vi "ThreeIncoming.vi"() -> ()   [LabVIEW 2019]
uses:
  <vilib>/rvi/Emulation/niFpgaGetClockAttributes.vi
  <vilib>/rvi/Emulation/niFpgaSctlEmulationGetInTimedLoop.vi
  <vilib>/rvi/Emulation/niFpgaEmulationReportErrorSimple.vi
  <vilib>/rvi/Emulation/niFpgaCriticalErrorInLSC.vi
  <vilib>/rvi/interface/RandomDataEmulation/niFpgaRandomDataHandleErrors.vi
  <vilib>/rvi/DataTransferAndStorage/Container/XNode/niFpgaContainer.xnode
  <vilib>/rvi/interface/RandomDataEmulation/nirviRandomDataFpgaReadWriteTemplate.vi
  <vilib>/Platform/TimedLoop/XDataNode/wakeup.ctl
  <vilib>/Platform/TimedLoop/XDataNode/XDNodeRunTimeDep.lvlib
  <vilib>/Platform/TimedLoop/XDataNode/nitl_modes.ctl
  <vilib>/Platform/TimedLoop/XDataNode/timing_clust.ctl
  <vilib>/Platform/TimedLoop/XDataNode/XDataNode.xnode
  SubModules/FPGA Addon Speciality IO/Source/Speciality FPGA IO.lvlib
  SubModules/FPGA Addon Speciality IO/Source/Types/QuadratureEncoder.Measure.Digital.Settings.ctl
  SubModules/FPGA Addon Speciality IO/Source/Types/QuadratureEncoder.Measure.Digital.Measurement.ctl
  SubModules/FPGA Addon Speciality IO/Source/Types/WSS.Generate.Digital.Settings.ctl
  SubModules/FPGA Addon Speciality IO/Source/Types/Static.Measure.Digital.Measurement.ctl
  SubModules/FPGA Addon Speciality IO/Source/Types/Static.Measure.Digital.Settings.ctl
  SubModules/FPGA Addon Speciality IO/Source/Types/Static.Generate.Digital.Settings.ctl
  SubModules/FPGA Addon Speciality IO/Source/Types/PWM.Generate.Digital.Settings.ctl
  SubModules/FPGA Addon Speciality IO/Source/Types/PWM.Measure.Digital.Settings.ctl
  SubModules/FPGA Addon Speciality IO/Source/Types/PWM.Measure.Digital.Measurement.ctl
panel:
  out "Measure.Digital.Ch0":T1={"ACTIVE TICKS"=4000, "INACTIVE TICKS"=12000, "ACQ TICKS"=1}
  out "Measure.Digital.Ch1":T1
  in  "Measure.Digital.Ch0.Settings":T2={"ACTIVE EDGE"=TRUE, "TIMEOUT"=40000000}
  in  "Measure.Digital.Ch1.Settings":T2={"ACTIVE EDGE"=FALSE, "TIMEOUT"=40000000}
  in  "Generate.Digital.Ch0.Internal.Settings":T3={"ACTIVE EDGE"=TRUE, "ACTIVE TICKS"=4000, "INACTIVE TICKS"=12000}
  in  "Generate.Digital.Ch1.Internal.Settings":T3={"ACTIVE EDGE"=FALSE, "ACTIVE TICKS"=60000000, "INACTIVE TICKS"=20000000}
  in  "Generate.Digital.Ch2.Internal.Settings":T4={"ACTIVE EDGE"=TRUE, "OUTPUT"=FALSE}
  in  "Measure.Digital.Ch2.Internal.Settings":T5={"ACTIVE EDGE"=TRUE}
  out "Measure.Digital.Ch2":T6
  in  "Generate.Digital.Ch3.Internal.Settings":T4={"ACTIVE EDGE"=TRUE, "OUTPUT"=FALSE}
  in  "Measure.Digital.Ch3.Internal.Settings":T5={"ACTIVE EDGE"=TRUE}
  out "Measure.Digital.Ch3":T6
  in  "Generate.Digital.Ch4.WSS.Settings":T7={"ACTIVE EDGE"=TRUE, "ACTIVE TICKS"=0, "INACTIVE TICKS"=0, "DATA"=0, "SENSOR TYPE"=0}
  out "Bit0":bool
  out "Bit1":bool
  out "Measurement.Digital.Ch5":T8
  in  "A":bool
  in  "B":bool
  in  "Z":bool
  in  "Measure.Digital.Ch5.QuadEncoder.Settings":T9={"DIRECTION"=0, "RESET VALUE"=0, "A RESET STATE"=TRUE, "B RESET STATE"=TRUE, "Z RESET STATE"=TRUE}
  in  "Group1.I16":i16
  in  "Group1.I8":i8
  in  "Group1.I64":i64
  in  "Group1.I32":i32
  in  "Group1.U16":u16
  in  "Group1.U8":u8
  in  "Group1.U64":u64
  in  "Group1.U32":u32
  in  "Group1.SGL":sgl
  in  "Group2.Boolean":bool
  out "Group1.I16 out":i16
  out "Group1.I8 out":i8
  out "Group1.I64 out":i64
  out "Group1.I32 out":i32
  out "Group1.U16 out":u16
  out "Group1.U8 out":u8
  out "Group1.U64 out":u64
  out "Group1.U32 out":u32
  out "Group1.SGL out":sgl
  out "Group2.Boolean out":bool
  in  "Group2.FXP24.5":fxp<+/-,24,5>
  in  "Group2.FXP16.5":fxp<+/-,16,5>
  in  "Group2.FXP32.8":fxp<+/-,32,8>
  in  "Group2.FXP64.32":fxp<+/-,64,32>
  out "Group2.FXP24.5 out":fxp<+/-,24,5>
  out "Group2.FXP16.5 out":fxp<+/-,16,5>
  out "Group2.FXP32.8 out":fxp<+/-,32,8>
  out "Group2.FXP64.32 out":fxp<+/-,64,32>
  in  "Group2.FXP16.7":fxp<+/-,16,7>
  out "Group2.FXP16.7 out":fxp<+/-,16,7>
  in  "Group2.FXP20.5":fxp<+/-,20,5>
  out "Group2.FXP20.5 out":fxp<+/-,20,5>
  in  "Group2.FXP27.5":fxp<+/-,27,5>
  out "Group2.FXP27.5 out":fxp<+/-,27,5>
  in  "Group2.FXP32.16":fxp<+/-,32,16>
  out "Group2.FXP32.16 out":fxp<+/-,32,16>
  in  "Group2.FXP16.3":fxp<+,16,3>
  out "Group2.FXP16.3 out":fxp<+,16,3>
  in  "Group2.FXP18.3":fxp<+,18,3>
  out "Group2.FXP18.3 out":fxp<+,18,3>
  in  "FXP18.3":fxp<+,18,3>
  out "FXP18.3 out":fxp<+,18,3>
  in  "FXP16.3":fxp<+,16,3>
  out "FXP16.3 out":fxp<+,16,3>
  in  "FXP32.16":fxp<+/-,32,16>
  out "FXP32.16 out":fxp<+/-,32,16>
  in  "FXP27.5":fxp<+/-,27,5>
  out "FXP27.5 out":fxp<+/-,27,5>
  in  "FXP20.5":fxp<+/-,20,5>
  out "FXP20.5 out":fxp<+/-,20,5>
  in  "FXP16.7":fxp<+/-,16,7>
  out "FXP16.7 out":fxp<+/-,16,7>
  out "FXP64.32 out":fxp<+/-,64,32>
  out "FXP32.8 out":fxp<+/-,32,8>
  out "FXP16.5 out":fxp<+/-,16,5>
  out "FXP24.5 out":fxp<+/-,24,5>
  in  "FXP64.32":fxp<+/-,64,32>
  in  "FXP32.8":fxp<+/-,32,8>
  in  "FXP16.5":fxp<+/-,16,5>
  in  "FXP24.5":fxp<+/-,24,5>
  out "Fast timeout":bool
  out "Med timeout":bool
  out "Slow timeout":bool
  in  "I16":i16
  in  "I8":i8
  in  "I64":i64
  in  "I32":i32
  in  "U16":u16
  in  "U8":u8
  in  "U64":u64
  in  "U32":u32
  in  "SGL":sgl
  in  "Boolean":bool
  out "I16 out":i16
  out "I8 out":i8
  out "I64 out":i64
  out "I32 out":i32
  out "U16 out":u16
  out "U8 out":u8
  out "U64 out":u64
  out "U32 out":u32
  out "SGL out":sgl
  out "Boolean out":bool
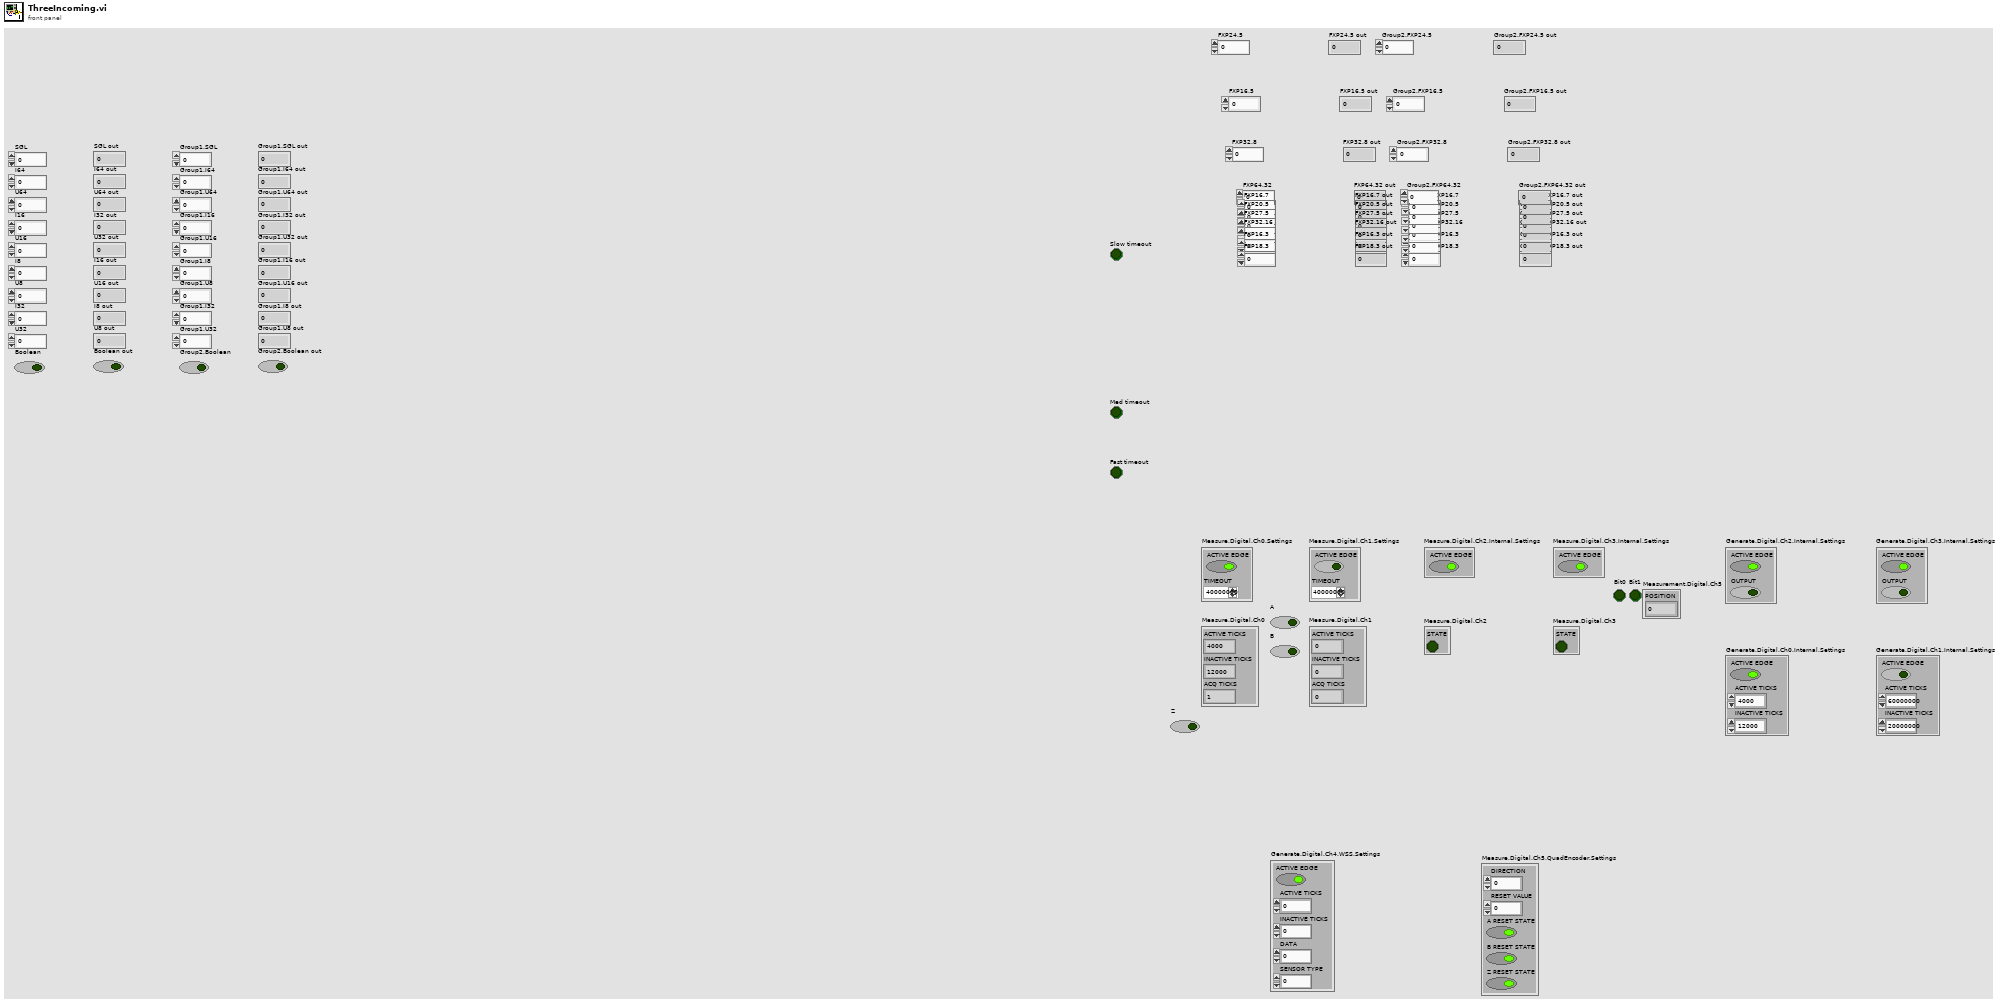
[diagram p1: front panel]
types:
  T1 = typedef "Speciality FPGA IO.lvlib/PWM.Measure.Digital.Measurement.ctl" = cluster{"ACTIVE TICKS":u32, "INACTIVE TICKS":u32, "ACQ TICKS":u32}
  T2 = typedef "Speciality FPGA IO.lvlib/PWM.Measure.Digital.Settings.ctl" = cluster{"ACTIVE EDGE":bool, "TIMEOUT":u32}
  T3 = typedef "Speciality FPGA IO.lvlib/PWM.Generate.Digital.Settings.ctl" = cluster{"ACTIVE EDGE":bool, "ACTIVE TICKS":u32, "INACTIVE TICKS":u32}
  T4 = typedef "Speciality FPGA IO.lvlib/Static.Generate.Digital.Settings.ctl" = cluster{"ACTIVE EDGE":bool, "OUTPUT":bool}
  T5 = typedef "Speciality FPGA IO.lvlib/Static.Measure.Digital.Settings.ctl" = cluster{"ACTIVE EDGE":bool}
  T6 = typedef "Speciality FPGA IO.lvlib/Static.Measure.Digital.Measurement.ctl" = cluster{"STATE":bool}
  T7 = typedef "Speciality FPGA IO.lvlib/WSS.Generate.Digital.Settings.ctl" = cluster{"ACTIVE EDGE":bool, "ACTIVE TICKS":u32, "INACTIVE TICKS":u32, "DATA":u8, "SENSOR TYPE":u8}
  T8 = typedef "Speciality FPGA IO.lvlib/QuadratureEncoder.Measure.Digital.Measurement.ctl" = cluster{"POSITION":i32}
  T9 = typedef "Speciality FPGA IO.lvlib/QuadratureEncoder.Measure.Digital.Settings.ctl" = cluster{"DIRECTION":u8, "RESET VALUE":i32, "A RESET STATE":bool, "B RESET STATE":bool, "Z RESET STATE":bool}
  T10 = typedef "XDNodeRunTimeDep.lvlib/timing_clust.ctl" = cluster{"Expected End [f-1]":u64, "Actual End [f-1]":u64, "Finished Late? [f-1]":bool, "Expected End [i-1]":u64, "Actual End [i-1]":u64, "Finished Late? [i-1]":bool, "Expected Start [i]":u64, "Actual Start [i]":u64, "Expected Start [f]":u64, "Actual Start [f]":u64, "Source Name":string, "Structure Name":string, "Period":i64, "Deadline":i64, "Offset":i64, "Start":i64, "Priority":i32, "Timeout":i32, "Mode":T11, "Wakeup Reason":T12, "Error":errorcluster, "Source Type":string, "Secondary Source Type":string, "Global End Time":u64, "Global Start Time":u64, "Frame Duration":u64, "Iteration Duration":u64, "Assigned CPU":i32, "I/O Scan Engine Mode":u32}
  T11 = typedef "XDNodeRunTimeDep.lvlib/nitl_modes.ctl" = enum32{"No Change", "Process missed periods, maintain original phase", "Discard missed periods, maintain original phase", "Process missed periods, ignore original phase", "Discard missed periods, ignore original phase"}
  T12 = typedef "XDNodeRunTimeDep.lvlib/wakeup.ctl" = enum32{"Normal", "Aborted", "Asynchronous wakeup", "Timing source error", "Timed loop error", "Timeout"}
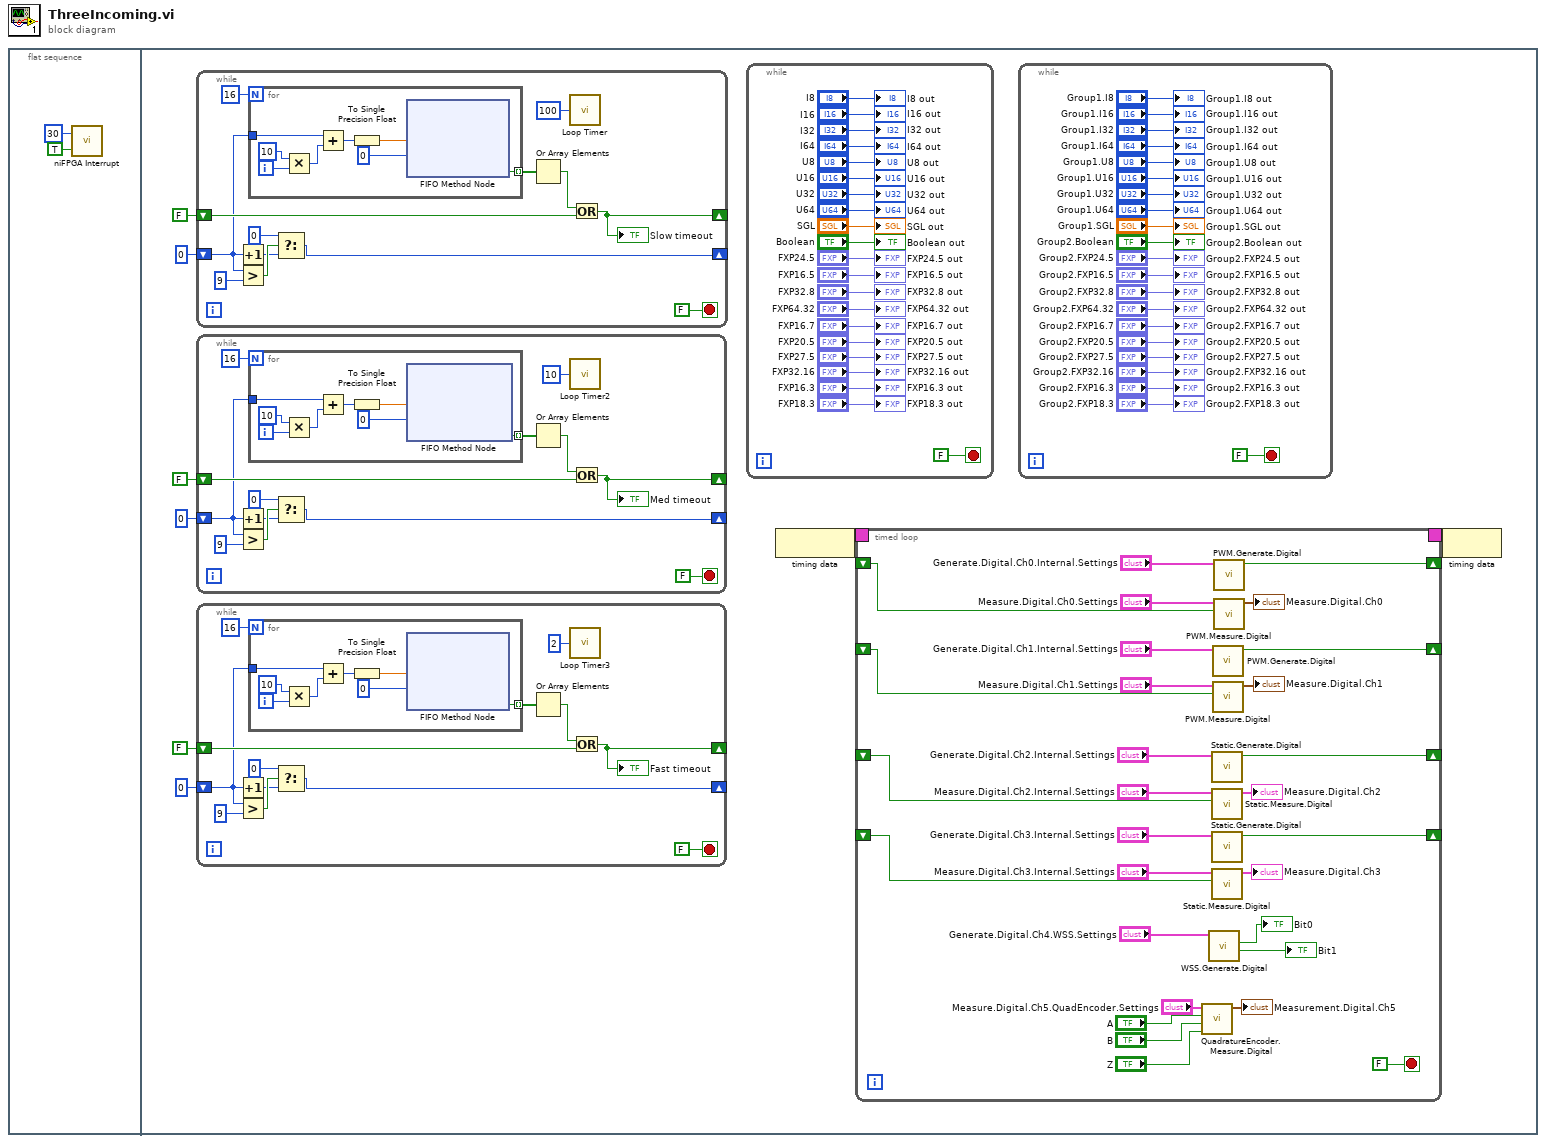
[diagram p0: block diagram]
diagram:
  n1 = flat-sequence {
    frame #0 {
      n2 = call <vilib>:"niFPGA Interrupt.vi"("Wait Until Cleared (F)"=TRUE, "IRQ Number (0)"=u8 30) -> ()  [unwired: 1 in]
    }
    frame #1 {
      n3 = while {
        shift-right: [w114] -> _
        shift-left: 0 ("t") -> [w107]
        shift-right: [w108] -> _
        shift-left: FALSE -> [w109]
        stop <- FALSE stop-if-true
        n4 = Increment(x=w107) -> (x+1=w112:i32)
        n5 = Greater?(x=w107, y=9) -> (0:w118:bool)
        n6 = for {
          N: 16 -> [_]
          tunnel: w107 -> [w127]
          tunnel: [w120] -> w111 mode=indexing
          i -> [w126]
          n7 = Multiply(x=10, y=w126) -> (x*y=w124:i32)
          n8 = Add(x=w127, y=w124) -> (x+y=w123:i32)
          n9 = To Single Precision Float(number=w123) -> (single precision float=w122:sgl)
          n10 = xnode ("FIFO Method Node")("Element"=w122, "Timeout"=0) -> ("Timed Out?"=w120:bool)  [unwired: 1 in, 1 out]
        }
        n11 = Select(t=0, s=w118, f=w112) -> (s? t:f=w114:i32)
        n12 = Or Array Elements(Boolean array=w111) -> (logical OR=w110:bool)
        n13 = call "Loop Timer"("Count(uSec)"=u32 100) -> ()  [unwired: 1 out]
        n14 = Or(x=w110, y=w109) -> (x .or. y?=w108:bool)
        "Slow timeout" <- w108
      }
      n15 = while {
        shift-right: [w93] -> _
        shift-left: 0 ("t") -> [w86]
        shift-right: [w87] -> _
        shift-left: FALSE -> [w88]
        stop <- FALSE stop-if-true
        n16 = Increment(x=w86) -> (x+1=w91:i32)
        n17 = Greater?(x=w86, y=9) -> (0:w97:bool)
        n18 = for {
          N: 16 -> [_]
          tunnel: w86 -> [w106]
          tunnel: [w99] -> w90 mode=indexing
          i -> [w105]
          n19 = Multiply(x=10, y=w105) -> (x*y=w103:i32)
          n20 = Add(x=w106, y=w103) -> (x+y=w102:i32)
          n21 = To Single Precision Float(number=w102) -> (single precision float=w101:sgl)
          n22 = xnode ("FIFO Method Node")("Element"=w101, "Timeout"=0) -> ("Timed Out?"=w99:bool)  [unwired: 1 in, 1 out]
        }
        n23 = Select(t=0, s=w97, f=w91) -> (s? t:f=w93:i32)
        n24 = Or Array Elements(Boolean array=w90) -> (logical OR=w89:bool)
        n25 = call "Loop Timer2"("Count(uSec)"=u32 10) -> ()  [unwired: 1 out]
        n26 = Or(x=w89, y=w88) -> (x .or. y?=w87:bool)
        "Med timeout" <- w87
      }
      n27 = while {
        shift-right: [w72] -> _
        shift-left: 0 ("t") -> [w65]
        shift-right: [w66] -> _
        shift-left: FALSE -> [w67]
        stop <- FALSE stop-if-true
        n28 = Increment(x=w65) -> (x+1=w70:i32)
        n29 = Greater?(x=w65, y=9) -> (0:w76:bool)
        n30 = for {
          N: 16 -> [_]
          tunnel: w65 -> [w85]
          tunnel: [w78] -> w69 mode=indexing
          i -> [w84]
          n31 = Multiply(x=10, y=w84) -> (x*y=w82:i32)
          n32 = Add(x=w85, y=w82) -> (x+y=w81:i32)
          n33 = To Single Precision Float(number=w81) -> (single precision float=w80:sgl)
          n34 = xnode ("FIFO Method Node")("Element"=w80, "Timeout"=0) -> ("Timed Out?"=w78:bool)  [unwired: 1 in, 1 out]
        }
        n35 = Select(t=0, s=w76, f=w70) -> (s? t:f=w72:i32)
        n36 = Or Array Elements(Boolean array=w69) -> (logical OR=w68:bool)
        n37 = call "Loop Timer3"("Count(uSec)"=u32 2) -> ()  [unwired: 1 out]
        n38 = Or(x=w68, y=w67) -> (x .or. y?=w66:bool)
        "Fast timeout" <- w66
      }
      n39 = while {
        stop <- FALSE stop-if-true
        "I16 out" <- "I16"
        "I8 out" <- "I8"
        "I64 out" <- "I64"
        "I32 out" <- "I32"
        "U16 out" <- "U16"
        "U8 out" <- "U8"
        "U64 out" <- "U64"
        "U32 out" <- "U32"
        "SGL out" <- "SGL"
        "Boolean out" <- "Boolean"
        "FXP24.5 out" <- "FXP24.5"
        "FXP16.5 out" <- "FXP16.5"
        "FXP32.8 out" <- "FXP32.8"
        "FXP64.32 out" <- "FXP64.32"
        "FXP16.7 out" <- "FXP16.7"
        "FXP20.5 out" <- "FXP20.5"
        "FXP27.5 out" <- "FXP27.5"
        "FXP32.16 out" <- "FXP32.16"
        "FXP16.3 out" <- "FXP16.3"
        "FXP18.3 out" <- "FXP18.3"
      }
      n40 = node-c288() -> (w4:T10)
      n41 = timed-loop {
        timing: w4 -> [_]
        timing-out: [_] -> w3
        shift-right: [w38] -> _
        shift-left: _ -> [w37]
        shift-right: [w36] -> _
        shift-left: _ -> [w35]
        shift-right: [w28] -> _
        shift-left: _ -> [w26]
        shift-right: [w19] -> _
        shift-left: _ -> [w21]
        stop <- FALSE stop-if-true
        n42 = call "QuadratureEncoder.Measure.Digital.vi"("Z"="Z", "B"="B", "A"="A", "Settings"="Measure.Digital.Ch5.QuadEncoder.Settings") -> ("Measurement"=→"Measurement.Digital.Ch5":T8)  [unwired: 7 in]
        n43 = call "WSS.Generate.Digital.vi"("Settings"="Generate.Digital.Ch4.WSS.Settings") -> ("Bit1"=→"Bit1":bool, "Bit0"=→"Bit0":bool)  [unwired: 8 in, 1 out]
        n44 = call "Static.Generate.Digital.vi"("Settings"="Generate.Digital.Ch2.Internal.Settings") -> ("Output"=w28:bool)  [unwired: 10 in]
        n45 = call "Static.Measure.Digital.vi"("State"=w26, "Settings"="Measure.Digital.Ch2.Internal.Settings") -> ("Measurement"=→"Measure.Digital.Ch2":T6)  [unwired: 9 in]
        n46 = call "Static.Generate.Digital.vi"("Settings"="Generate.Digital.Ch3.Internal.Settings") -> ("Output"=w19:bool)  [unwired: 10 in]
        n47 = call "Static.Measure.Digital.vi"("State"=w21, "Settings"="Measure.Digital.Ch3.Internal.Settings") -> ("Measurement"=→"Measure.Digital.Ch3":T6)  [unwired: 9 in]
        n48 = call "PWM.Generate.Digital.vi"("Settings"="Generate.Digital.Ch1.Internal.Settings") -> ("Output"=w38:bool)  [unwired: 10 in]
        n49 = call "PWM.Measure.Digital.vi"("State"=w37, "Settings"="Measure.Digital.Ch1.Settings") -> ("Measurement"=→"Measure.Digital.Ch1":T1)  [unwired: 8 in, 1 out]
        n50 = call "PWM.Generate.Digital.vi"("Settings"="Generate.Digital.Ch0.Internal.Settings") -> ("Output"=w36:bool)  [unwired: 10 in]
        n51 = call "PWM.Measure.Digital.vi"("State"=w35, "Settings"="Measure.Digital.Ch0.Settings") -> ("Measurement"=→"Measure.Digital.Ch0":T1)  [unwired: 8 in, 1 out]
      }
      n52 = while {
        stop <- FALSE stop-if-true
        "Group1.I16 out" <- "Group1.I16"
        "Group1.I8 out" <- "Group1.I8"
        "Group1.I64 out" <- "Group1.I64"
        "Group1.I32 out" <- "Group1.I32"
        "Group1.U16 out" <- "Group1.U16"
        "Group1.U8 out" <- "Group1.U8"
        "Group1.U64 out" <- "Group1.U64"
        "Group1.U32 out" <- "Group1.U32"
        "Group1.SGL out" <- "Group1.SGL"
        "Group2.Boolean out" <- "Group2.Boolean"
        "Group2.FXP24.5 out" <- "Group2.FXP24.5"
        "Group2.FXP16.5 out" <- "Group2.FXP16.5"
        "Group2.FXP32.8 out" <- "Group2.FXP32.8"
        "Group2.FXP64.32 out" <- "Group2.FXP64.32"
        "Group2.FXP16.7 out" <- "Group2.FXP16.7"
        "Group2.FXP20.5 out" <- "Group2.FXP20.5"
        "Group2.FXP27.5 out" <- "Group2.FXP27.5"
        "Group2.FXP32.16 out" <- "Group2.FXP32.16"
        "Group2.FXP16.3 out" <- "Group2.FXP16.3"
        "Group2.FXP18.3 out" <- "Group2.FXP18.3"
      }
      n53 = node-c288(w3) -> ()
    }
  }
